vi "IDS Initialize Camera.vi"(0 "Camera ID":refnum<k24>, 7 "IDS Cam Img Ref":T1) -> (8 "IDS Cam Img Ref":T1, 15 "Error Out":errorcluster)   [LabVIEW 2025]
uses:
  C:/Users/Photonics03/Documents/Microscope-Control/Device Library/Cameras/IDS/IDS LabView Examples/LabVIEW/ueye.NET/uEyeDotNet.dll
  IDS LabView Examples/LabVIEW/ueye.NET/uEyeDotNet.dll
  <vilib>/vision/Image Controls.llb/IMAQ Image.ctl
  Camera Controls/Camera IMAQ Key Info.ctl
panel:
  out "s32Value":i32
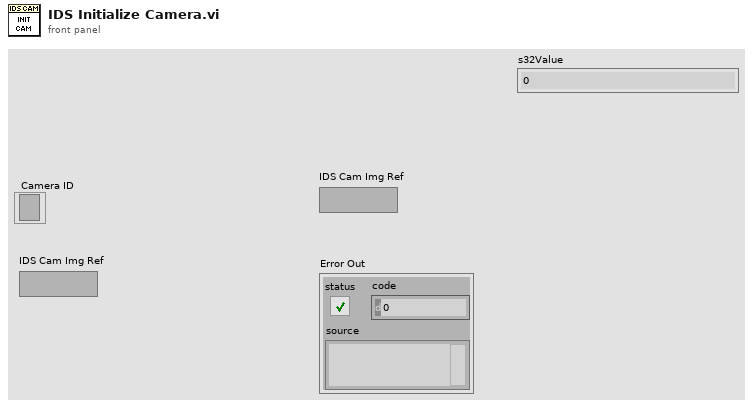
[diagram p1: front panel]
types:
  T1 = typedef "IMAQ Image.ctl" = refnum<image>
  T2 = typedef "Camera IMAQ Key Info.ctl" = cluster{"Frame":u32, "Sensor Height":i32, "Sensor Width":i32, "ROI Height":i32, "ROI Width":i32, "ROI Enable?":bool, "Bit per Pixel":u8}
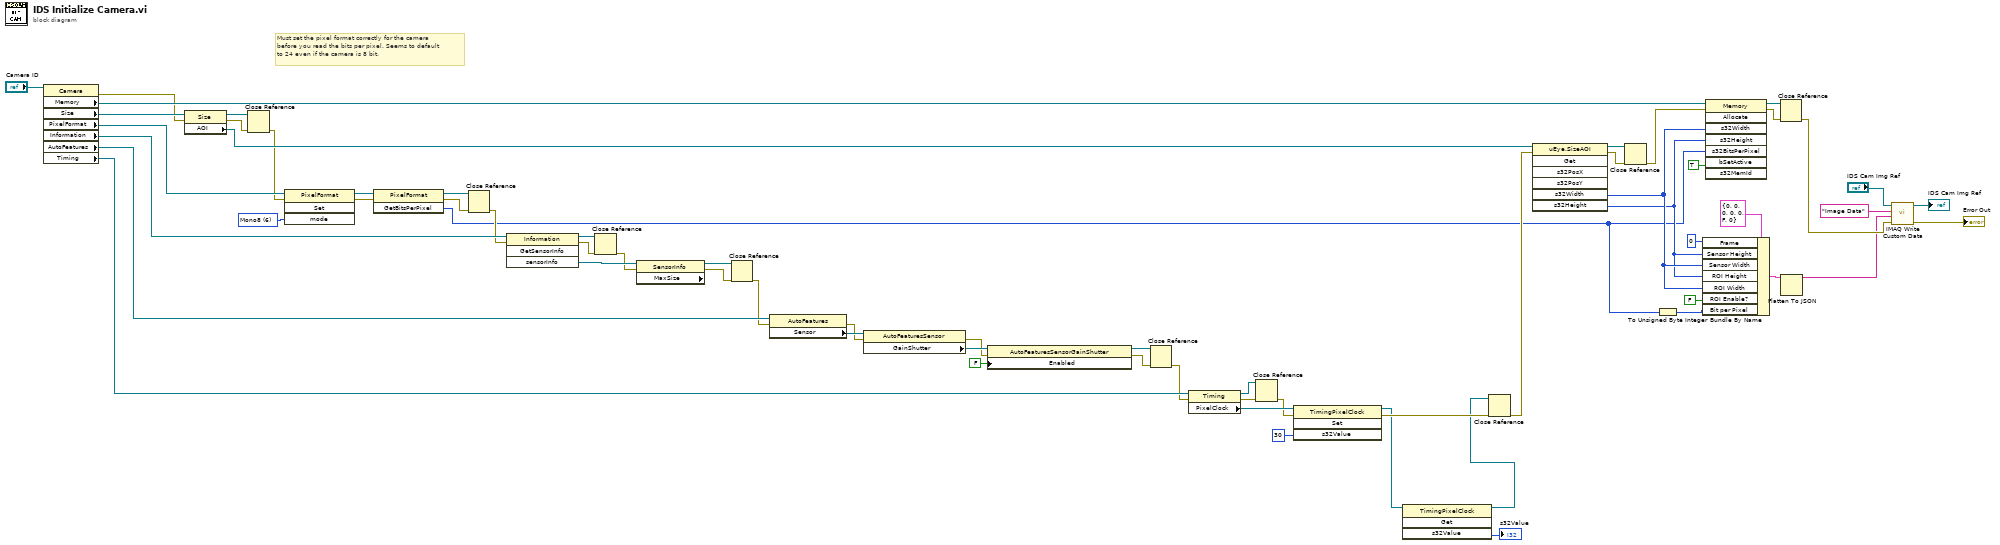
[diagram p0: block diagram]
diagram:
  w31 = 6 items=["BGRA8Packed"=0, "BGR8Packed"=1, "BGR565Packed"=2, "BGR5Packed"=3, "Mono8"=6, "SensorRaw8"=11, "UYVYPacked"=12, "UYVYMonoPacked"=13, "UYVYBayerPacked"=14, "CBYCRYPacked"=23, "BGRY8Packed"=24, "BGR10Packed"=25, "Mono12"=26, "SensorRaw12"=27, "Mono16"=28, "SensorRaw16"=29, "BGR12Unpacked"=30, "BGRA12Unpacked"=31, "Jpeg"=32, "SensorRaw10"=33, "Mono10"=34, "BGR10Unpacked"=35, "RGBA8Packed"=128, "RGB8Packed"=129, "RGBY8Packed"=152, "RGB10Packed"=153, "RGB12Unpacked"=158, "RGBA12Unpacked"=159, "RGB10Unpacked"=163, "RGB8Planar"=8321, "PreferPackedSourceFormat"=16384] ("mode")
  # "Must set the pixel format correctly for the camera\nbefore you read the bits per pixel. Seems to default\nto 24 even if the camera is 8 bit."
  n1 = property class="Camera"(reference="Camera ID") -> (error out=w52:errorcluster, "Memory"=w60:refnum<k24>, "Size"=w54:refnum<k24>, "PixelFormat"=w28:refnum<k24>, "Information"=w57:refnum<k24>, "AutoFeatures"=w39:refnum<k24>, "Timing"=w23:refnum<k24>)  [unwired: 1 in, 1 out]
  n2 = property class="Size"(reference=w54, error in=w52) -> (reference out=w62:refnum<k24>, error out=w51:errorcluster, "AOI"=w63:refnum<k24>)
  n3 = Close Reference(reference=w62, error in (no error)=w51) -> (error out=w27:errorcluster)
  n4 = invoke class="PixelFormat" method="Set"(reference=w28, error in=w27, "mode"=w31) -> (reference out=w26:refnum<k24>, error out=w25:errorcluster)  [unwired: 1 in, 2 out]
  n5 = invoke class="PixelFormat" method="GetBitsPerPixel"(reference=w26, error in=w25) -> (reference out=w29:refnum<k24>, error out=w50:errorcluster, "GetBitsPerPixel"=w5:i32)  [unwired: 1 in]
  n6 = Close Reference(reference=w29, error in (no error)=w50) -> (error out=w49:errorcluster)
  n7 = invoke class="Information" method="GetSensorInfo"(reference=w57, error in=w49) -> (reference out=w30:refnum<k24>, error out=w48:errorcluster, "sensorInfo"=w56:refnum<k24>)  [unwired: 2 in, 1 out]
  n8 = Close Reference(reference=w30, error in (no error)=w48) -> (error out=w46:errorcluster)
  n9 = property class="SensorInfo" props=["MaxSize"](reference=w56, error in=w46) -> (reference out=w55:refnum<k24>, error out=w47:errorcluster)  [unwired: 1 out]
  n10 = Close Reference(reference=w55, error in (no error)=w47) -> (error out=w24:errorcluster)
  n11 = property class="AutoFeatures"(reference=w39, error in=w24) -> (error out=w34:errorcluster, "Sensor"=w38:refnum<k24>)  [unwired: 1 out]
  n12 = property class="AutoFeaturesSensor"(reference=w38, error in=w34) -> (error out=w35:errorcluster, "GainShutter"=w37:refnum<k24>)  [unwired: 1 out]
  n13 = property class="AutoFeaturesSensorGainShutter"(reference=w37, error in=w35, "Enabled"=FALSE) -> (reference out=w33:refnum<k24>, error out=w32:errorcluster)
  n14 = Close Reference(reference=w33, error in (no error)=w32) -> (error out=w21:errorcluster)
  n15 = property class="Timing"(reference=w23, error in=w21) -> (reference out=w18:refnum<k24>, error out=w19:errorcluster, "PixelClock"=w22:refnum<k24>)
  n16 = Close Reference(reference=w18, error in (no error)=w19) -> (error out=w17:errorcluster)
  n17 = invoke class="TimingPixelClock" method="Set"(reference=w22, error in=w17, "s32Value"=30) -> (reference out=w3:refnum<k24>, error out=w20:errorcluster)  [unwired: 1 in, 2 out]
  n18 = invoke class="TimingPixelClock" method="Get"(reference=w3) -> (reference out=w2:refnum<k24>, "s32Value"=→"s32Value":i32)  [unwired: 3 in, 2 out]
  n19 = Close Reference(reference=w2, error in (no error)=w20) -> (error out=w15:errorcluster)
  n20 = invoke class="uEye.SizeAOI" method="Get"(reference=w63, error in=w15) -> (reference out=w61:refnum<k24>, error out=w45:errorcluster, "s32Width"=w7:i32, "s32Height"=w6:i32)  [unwired: 5 in, 3 out]
  n21 = Close Reference(reference=w61, error in (no error)=w45) -> (error out=w44:errorcluster)
  n22 = To Unsigned Byte Integer(number=w5) -> (unsigned 8bit integer=w4:u8)
  n23 = Bundle By Name(cluster=T2 {"Frame"=0, "Sensor Height"=0, "Sensor Width"=0, "ROI Height"=0, "ROI Width"=0, "ROI Enable?"=FALSE, "Bit per Pixel"=0} ("Camera IMAQ Key Info"), "Frame"=u32 0, "Sensor Height"=w6, "Sensor Width"=w7, "ROI Height"=w6, "ROI Width"=w7, "ROI Enable?"=FALSE, "Bit per Pixel"=w4) -> (w12:T2)
  n24 = invoke class="Memory" method="Allocate"(reference=w60, error in=w44, "s32Width"=w7, "s32Height"=w6, "s32BitsPerPixel"=w5, "bSetActive"=TRUE) -> (reference out=w58:refnum<k24>, error out=w43:errorcluster)  [unwired: 2 in, 6 out]
  n25 = Close Reference(reference=w58, error in (no error)=w43) -> (error out=w42:errorcluster)
  n26 = Flatten To JSON(anything=w12) -> (JSON string=w11:string)  [unwired: 2 in, 1 out]
  n27 = call "IMAQ Write Custom Data"("error in (no error)"=w42, "Custom Data In"=w11, "Key"="Image Data", "Image"="IDS Cam Img Ref") -> ("error out"=→"Error Out":errorcluster, "Image Out"=→"IDS Cam Img Ref":T1)  [unwired: 6 in]
